vi "POI Gen Engine.vi"(9 "Function":T1) -> (2 "empty?":bool)   [LabVIEW 2020]
uses:
  Typedefs/Duplicate POI function enum.ctl
  <vilib>/vision/Image Controls.llb/IMAQ Image.ctl
  Typedefs/ROI ID Enum.ctl
  Typedefs/Redraw ROI.ctl
  Typedefs/ROI management FG states.ctl
  Globals/gl_ROI Entry UI globals.vi
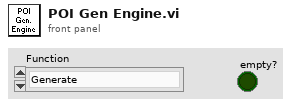
[diagram p1: front panel]
types:
  T1 = typedef "Duplicate POI function enum.ctl" = enum16{"Generate", "Adjust number of POI", "Clear register"}
  T2 = typedef "IMAQ Image.ctl" = refnum<image>
  T3 = typedef "ROI entry screen ctrl refs cluster.ctl" = cluster{"Done button":refnum<vi>, "Imaging button":refnum<vi>, "Acquisition button":refnum<vi>, "Scan dwell time per pixel (us)":refnum<vi>, "# of planes":refnum<vi>, "Zoom Ctrl":refnum<vi>, "Equal size":refnum<vi>, "Channel":refnum<vi>, "Image Display":refnum<vi>, "Z-Plane Selector":refnum<vi>, "Number of lines left":refnum<vi>, "Z-stack folder path":refnum<vi>, "POI Density":refnum<vi>, "Arb Plane Entry":refnum<vi>, "Whole Plane":refnum<vi>, "Line Mode":refnum<vi>, "Clear Last":refnum<vi>, "Clear All":refnum<vi>, "Delete Lines":refnum<vi>, "Trial Length (sec)":refnum<vi>, "Palette Type":refnum<vi>, "Intensity slider":refnum<vi>, "# POI":refnum<vi>, "Max Z Proj":refnum<vi>, "Zplane ind":refnum<vi>, "Wavelength (nm)":refnum<vi>, "Number of Trials":refnum<vi>, "Funct stim.trig.enable":refnum<vi>, "Funct stim.trig.delay (s)":refnum<vi>, "Line Mode":refnum<vi>, "Step size (µm)":refnum<vi>, "ROI move mode":refnum<vi>, "Cool-down time (s)":refnum<vi>, "Enable cool-down time":refnum<vi>, "Motor Z ind. (um)":refnum<vi>, "AOL Z ind. (um)":refnum<vi>, "Load Reference Image":refnum<vi>, "Rel.  Res.":refnum<vi>, "ROI LIST":refnum<vi>, "Show All":refnum<vi>, "ROI Type":refnum<vi>, "Start Plane":refnum<vi>, "Stop Plane":refnum<vi>, "Offset ROI":refnum<vi>, "Tab Control":refnum<vi>, "Laser Power(%)":refnum<vi>, "Cycle rate":refnum<vi>, "FOV (Ind.)":refnum<vi>, "Frame Size (Ind.)":refnum<vi>, "Resolution (Ind.)":refnum<vi>, "Pixel Density (Ind)":refnum<vi>, "Laser Power (Ind.)":refnum<vi>, "Dwell Time (Ind.)":refnum<vi>, "Adj MC":refnum<vi>}
  T4 = cluster{"Global Rectangle":i32[], "Contours":cluster{"Contour Type":u32, "ROI Type":u32, "Points":i32[]}[]}
  T5 = typedef "ROI management FG states.ctl" = enum16{"Read", "Write", "Write-from dataset", "Clear Last", "Clear All", "Delete ROI", "Update ROIs time", "Reload last ROI set", "Modify ROI Parameters", "Offset all ROI", "Offset visible ROI", "Modify Dwell Time", "Modify Laser Power"}
  T6 = typedef "Redraw ROI.ctl" = enum16{"Redraw All", "Redraw Deselected", "Draw Last", "Redraw Selected"}
  T7 = typedef "ROI ID Enum.ctl" = enum16{"Point", "MiniScan", "Comp. MiniScan", "Rectangle", "Comp. volume", "Arb. plane point", "None"}
  T8 = cluster{"Pos. X":i32, "Pos. Y":i32, "Radius":i32, "Core Area":i32}[]
  T9 = typedef "ROI Z-stack settings info.ctl" = cluster{"Zoom":dbl, "POI Dwell time":dbl, "Rel. Res":dbl, "Laser Power %":dbl, "Frame Size":dbl, "FOV":dbl}
  T10 = typedef "ROI spec.ctl" = cluster{"ROI Enum":T7, "Coordinates":i32[], "Zoom":dbl, "POI Dwell time":dbl, "Rel. Resolution":dbl, "Laser Power":dbl, "Frame Size":dbl, "FOV":dbl, "Z start":dbl, "Z stop":dbl, "Z planeIdx(s)":i32[], "Z planecodes(s)":u8[]}
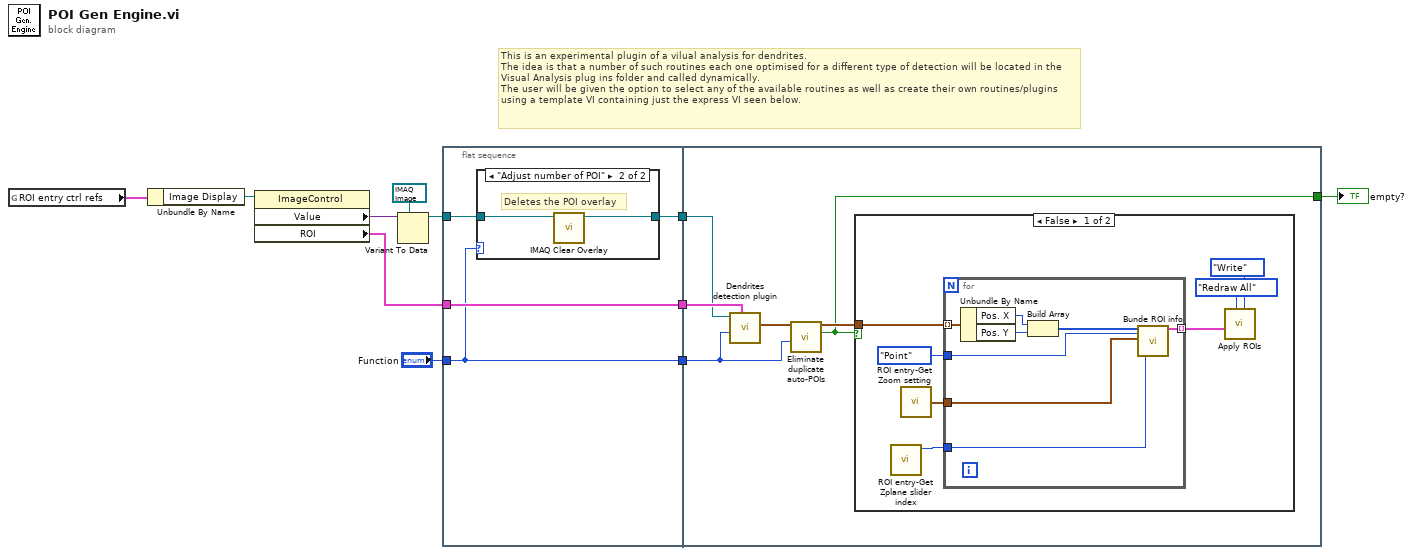
[diagram p0: block diagram]
diagram:
  # "This is an experimental plugin of a vilual analysis for dendrites.\nThe idea is that a number of such routines each one optimised for a different type of detection will be located in the Visual Analysis plug ins folder and called dynamically.\nThe user will be given the option to select any of the available routines as well as create their own routines/plugins using a template VI containing just the express VI seen below."
  n1 = global read "gl_ROI Entry UI globals.vi" "ROI entry ctrl refs"() -> (w1:T3)
  n2 = Unbundle By Name(w1) -> ("Image Display"=w6:refnum<vi>)
  n3 = property class="ImageControl"(reference=w6) -> ("Value"=w5:variant, "ROI"=w2:T4)  [unwired: 1 in, 2 out]
  n4 = Variant To Data(type=T2 refnum ("Image ref in"), Variant=w5) -> (data=w3:T2)  [unwired: 1 in, 1 out]
  n5 = flat-sequence {
    tunnel: "Function" -> [w12]
    tunnel: [w12] -> w11
    tunnel: w2 -> [w15]
    tunnel: [w15] -> w10
    tunnel: [w13] -> w9
    tunnel: w3 -> [w14]
    tunnel: w11 -> [w20]
    tunnel: w10 -> [w22]
    tunnel: w9 -> [w21]
    tunnel: [w19] -> w8
    frame #0 {
      n6 = case shown="\"Adjust number of POI\"" w12 {
        tunnel: w14 -> [w16 w18]
        tunnel: [w16 w17] -> w13
        frame "Generate", Default {
        }
        frame "Adjust number of POI" {
          # "Deletes the POI overlay"
          n7 = call "IMAQ Clear Overlay"("Image"=w18) -> ("Image Out"=w17:T2)  [unwired: 9 in, 1 out]
        }
      }
    }
    frame #1 {
      n8 = call "Dendrites detection plugin.vi"("ROI"=w22, "Function"=w20, "16 bit image in"=w21) -> ("Circles Data"=w23:T8)  [unwired: 5 in, 3 out]
      n9 = call "Eliminate duplicate auto-POIs.vi"("Function"=w20, "Circles Data in"=w23) -> ("empty?"=w19:bool, "Circles Data out"=w24:T8)  [unwired: 8 in]
      n10 = case shown="False" w19 {
        tunnel: w24 -> [w31 _]
        frame False {
          n11 = call "ROI entry-Get Zplane slider index.vi"() -> ("Z-plane slider's index (zero-based)"=w27:i32)  [unwired: 10 in, 1 out]
          n12 = call "ROI entry-Get Zoom setting.vi"() -> ("AOLZ Settings"=w25:T9)  [unwired: 7 in, 8 out]
          n13 = for {
            tunnel: w31 -> [w37] mode=indexing
            tunnel: [w35] -> w30 mode=indexing
            tunnel: ROI_ID_Enum."Point" ("ROI Enum") -> [w34]
            tunnel: w27 -> [w33]
            tunnel: w25 -> [w32]
            n14 = Unbundle By Name(w37) -> ("Pos. X"=w38:i32, "Pos. Y"=w39:i32)
            n15 = Build Array(w38, w39) -> (w36:i32[])
            n16 = call "Bunde ROI info.vi"("ROI Coordinates"=w36, "ROI Enum"=w34, "Z stack Settings"=w32, "ZplaneIndex"=w33) -> ("ROI Info"=w35:T10)  [unwired: 15 in]
          }
          n17 = call "Apply ROIs.vi"("Function"=ROI_management_FG_states."Write", "Mode (Redraw All)"=Redraw_ROI."Redraw All", "ROIs Info []"=w30) -> ()  [unwired: 6 in, 3 out]
        }
        frame True {
        }
      }
    }
  }
  "empty?" <- w8
